vi "DAQ.Init.vi"(8 "error in (no error)":errorcluster, 11 "DAQmx.AO in":refnum<class "DAQmx.AO.lvclass">) -> (0 "error out":errorcluster, 3 "DAQmx.AO out":refnum<class "DAQmx.AO.lvclass">)   [LabVIEW 2016, in "DAQmx.AO.lvclass"]
uses:
  DAQmx.AO.lvclass
  C:/user/patrick/hg/levy_inst_lockin/src/SMOs/DAQ/DAQ.lvclass
  C:/user/patrick/hg/levy_inst_lockin/src/SMOs/DAQmx/DAQmx.lvclass
  DAQ/DAQ.lvclass/DAQ.ctl
  DAQmx/DAQmx.lvclass/DAQmx.ctl
  DAQmx.AO.lvclass/DAQmx.AO.ctl
  <vilib>/DAQmx/create/channels.llb/DAQmx Create Channel (AO-Voltage-Basic).vi
  <vilib>/DAQmx/configure/timing.llb/DAQmx Timing (Sample Clock).vi
  <resource>/objmgr/daqmx.rc
  DAQ/DAQ.lvclass
  DAQmx/DAQmx.lvclass
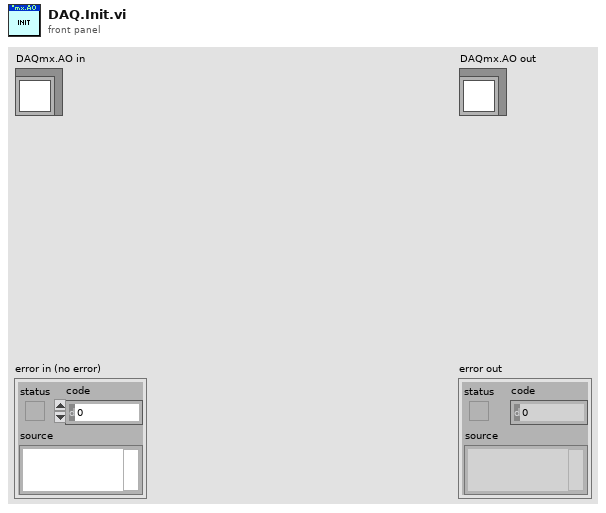
[diagram p1: front panel]
types:
  T1 = typedef "DAQ.lvclass/DAQ_Config.ctl" = cluster{"Channels":T2, "DAQ_Type":T3, "minimum value":dbl, "maximum value":dbl, "DAQ_SamplingInfo":T4, "DAQ_SamplingMode":T5}
  T2 = typedef "DAQ.lvclass/PrivateEvents--DAQ.AI.Channels.ctl" = string
  T3 = typedef "DAQ.lvclass/DAQ_Type.ctl" = enum16{"AI", "AO"}
  T4 = typedef "DAQ.lvclass/DAQ_SamplingInfo.ctl" = cluster{"Fs":dbl, "#s":i32}
  T5 = typedef "DAQ.lvclass/DAQ_SamplingMode.ctl" = enum16{"Continuous", "Finite"}
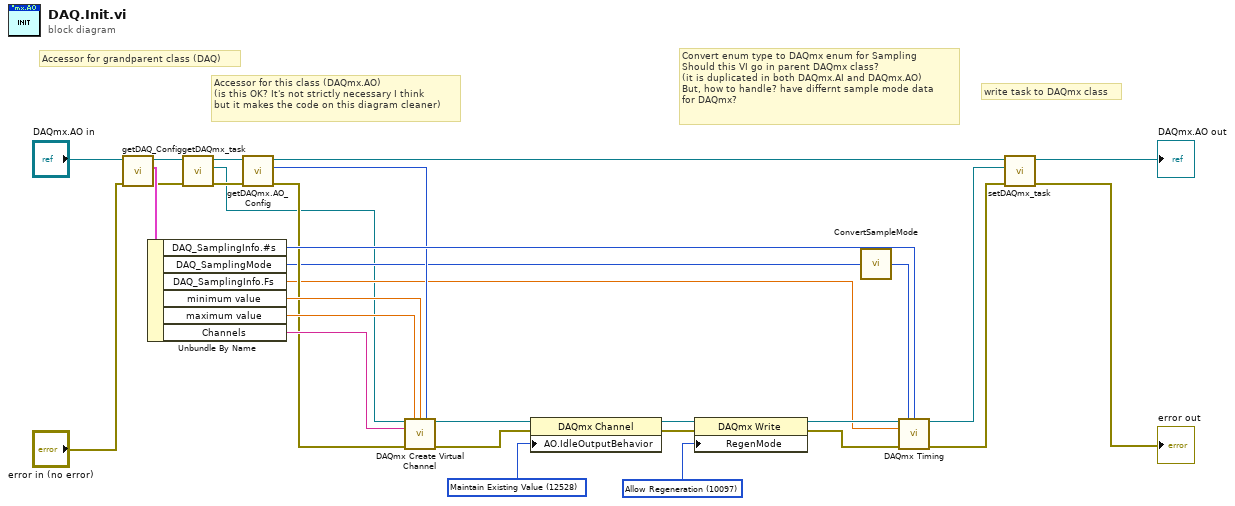
[diagram p0: block diagram]
diagram:
  w29 = 10097 items=["Allow Regeneration"=10097, "Do Not Allow Regeneration"=10158] ("RegenMode")
  w30 = 12528 items=["Zero Volts"=12526, "High-Impedance"=12527, "Maintain Existing Value"=12528] ("AO.IdleOutputBehavior")
  # "write task to DAQmx class"
  # "Accessor for this class (DAQmx.AO)\n(is this OK? It's not strictly necessary I think\nbut it makes the code on this diagram cleaner)"
  # "Accessor for grandparent class (DAQ)"
  # "Convert enum type to DAQmx enum for Sampling\nShould this VI go in parent DAQmx class?\n(it is duplicated in both DAQmx.AI and DAQmx.AO)\nBut, how to handle? have differnt sample mode data\nfor DAQmx?"
  n1 = call "getDAQ_Config.vi"("error in (no error)"="error in (no error)", "DAQ in"="DAQmx.AO in") -> ("error out"=w6:errorcluster, "DAQ_Config"=w21:T1, "DAQ out"=w7:refnum<class "DAQmx.AO.lvclass">)  [unwired: 7 in]
  n2 = Unbundle By Name(w21) -> ("DAQ_SamplingInfo.#s"=w17:i32, "DAQ_SamplingMode"=w10:T5, "DAQ_SamplingInfo.Fs"=w8:dbl, "minimum value"=w20:dbl, "maximum value"=w19:dbl, "Channels"=w18:T2)
  n3 = call "getDAQmx_task.vi"("error in (no error)"=w6, "DAQmx in"=w7) -> ("error out"=w5:errorcluster, "task"=w3:refnum<k21>, "DAQmx out"=w4:refnum<class "DAQmx.AO.lvclass">)  [unwired: 7 in]
  n4 = call "getDAQmx.AO_Config.vi"("error in (no error)"=w5, "DAQmx.AO in"=w4) -> ("error out"=w11:errorcluster, "output terminal configuration"=w13:i32, "DAQmx.AO out"=w12:refnum<class "DAQmx.AO.lvclass">)  [unwired: 7 in]
  n5 = call-poly <vilib>:"DAQmx Create Virtual Channel.vi"("task in"=w3, "maximum value"=w19, "minimum value"=w20, "output terminal configuration"=w13, "physical channels"=w18, "error in"=w11) -> ("task out"=w26:refnum<k21>, "error out"=w25:errorcluster)  [unwired: 8 in]
  n6 = property class="DAQmx Channel"(reference=w26, error in=w25, "AO.IdleOutputBehavior"=w30) -> (reference out=w24:refnum<k21>, error out=w23:errorcluster)
  n7 = property class="DAQmx Write"(reference=w24, error in=w23, "RegenMode"=w29) -> (reference out=w28:refnum<k21>, error out=w27:errorcluster)
  n8 = call "ConvertSampleMode.vi"("SamplingMode"=w10) -> ("sample mode"=w9:i32)
  n9 = call-poly <vilib>:"DAQmx Timing.vi"("task/channels in"=w28, "sample mode"=w9, "samples per channel"=w17, "rate"=w8, "error in"=w27) -> ("task out"=w16:refnum<k21>, "error out"=w15:errorcluster)  [unwired: 9 in]
  n10 = call "setDAQmx_task.vi"("error in (no error)"=w15, "task"=w16, "DAQmx in"=w12) -> ("error out"=→"error out":errorcluster, "DAQmx out"=→"DAQmx.AO out":refnum<class "DAQmx.AO.lvclass">)  [unwired: 7 in]
